vi "_Update Range Index.vi"(7 "Refrence":T1, 11 "XScale.Range in":T1) -> (3 "XScale.Range out":T1)   [LabVIEW 2017, in "XTriPhaseGraph.xctl"]
uses:
  XTriPhaseGraph.xctl
  <vilib>/Utility/miscctls.llb/LVRangeTypeDef.ctl
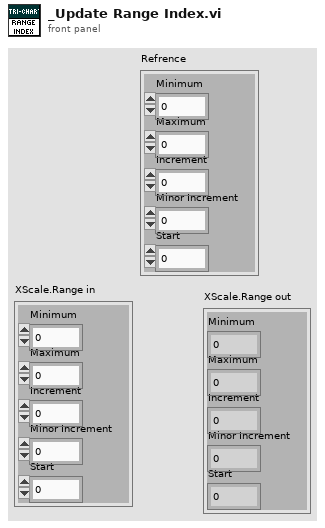
[diagram p1: front panel]
types:
  T1 = typedef "LVRangeTypeDef.ctl" = cluster{"Minimum":dbl, "Maximum":dbl, "Increment":dbl, "Minor Increment":dbl, "Start":dbl}
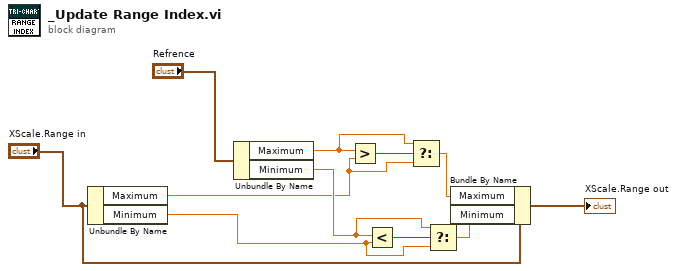
[diagram p0: block diagram]
diagram:
  n1 = Unbundle By Name("XScale.Range in") -> ("Maximum"=w4:dbl, "Minimum"=w7:dbl)
  n2 = Unbundle By Name("Refrence") -> ("Maximum"=w3:dbl, "Minimum"=w6:dbl)
  n3 = Greater?(x=w3, y=w4) -> (0:w2:bool)
  n4 = Less?(x=w6, y=w7) -> (x < y?=w5:bool)
  n5 = Select(t=w3, s=w2, f=w4) -> (s? t:f=w10:dbl)
  n6 = Select(t=w6, s=w5, f=w7) -> (s? t:f=w8:dbl)
  n7 = Bundle By Name(cluster="XScale.Range in", "Maximum"=w10, "Minimum"=w8) -> (→"XScale.Range out":T1)
